vi "Apply Arm Motor Limits.vi"(8 "error in (no error)":errorcluster, 11 "KUKA youBot arm in":refnum<class "NI_Robotics_KUKA youBot Arm.lvclass">) -> (0 "error out":errorcluster, 3 "KUKA youBot arm out":refnum<class "NI_Robotics_KUKA youBot Arm.lvclass">)   [LabVIEW 2017, in "NI_Robotics_KUKA youBot Host.lvlib" / "NI_Robotics_KUKA youBot Arm.lvclass"]
uses:
  <vilib>/robotics/KUKA youBot/Basic Device/Arm/NI_Robotics_KUKA youBot Arm.lvclass
  <vilib>/robotics/KUKA youBot/Basic Device/Arm/NI_Robotics_KUKA youBot Arm.lvclass/NI_Robotics_KUKA youBot Arm.ctl
  <vilib>/robotics/KUKA youBot/Motor/Arm Motor/NI_Robotics_KUKA youBot Arm Motor.lvclass
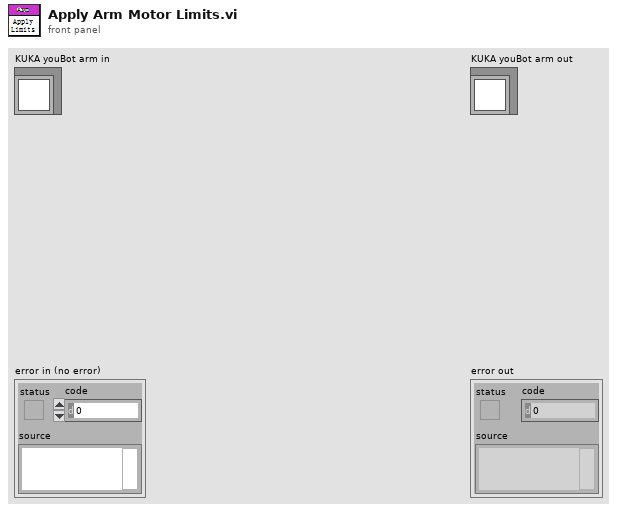
[diagram p1: front panel]
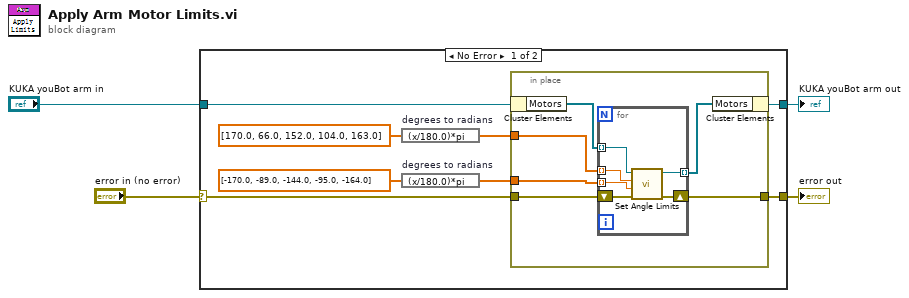
[diagram p0: block diagram]
diagram:
  n1 = case shown="No Error" "error in (no error)" {
    selector: "error in (no error)" -> [w11 w25]
    tunnel: [w10 w25] -> w3
    tunnel: [w9 w26] -> w1
    tunnel: "KUKA youBot arm in" -> [w12 w26]
    frame No Error {
      n2 = expression code="(x/180.0)*pi" "degrees to radians"(dbl[] [170.0, 66.0, 152.0, 104.0, 163.0]) -> (w6:dbl[])
      n3 = expression code="(x/180.0)*pi" "degrees to radians"(dbl[] [-170.0, -89.0, -144.0, -95.0, -164.0]) -> (w5:dbl[])
      n4 = in-place {
        in-place-border: w11 -> [w16]
        in-place-border: [w15] -> w10
        in-place-border: w6 -> [w14]
        in-place-border: w5 -> [w13]
        n5 = in-place-cluster #1(w12) -> ("Motors"=w18:refnum<class "NI_Robotics_KUKA youBot Arm Motor.lvclass">[])
        n6 = for {
          tunnel: w18 -> [w24] mode=indexing
          tunnel: [w23] -> w17 mode=indexing
          shift-right: [w21] -> w15
          shift-left: w16 -> [w22]
          tunnel: w14 -> [w20] mode=indexing
          tunnel: w13 -> [w19] mode=indexing
          n7 = call <vilib>:"Set Angle Limits.vi"("error in (no error)"=w22, "min angle (rad)"=w19, "max angle (rad)"=w20, "KUKA youBot arm motor in"=w24) -> ("error out"=w21:errorcluster, "KUKA youBot arm motor out"=w23:refnum<class "NI_Robotics_KUKA youBot Arm Motor.lvclass">)  [unwired: 6 in]
        }
        n8 = in-place-cluster #1("Motors"=w17) -> (w9:refnum<class "NI_Robotics_KUKA youBot Arm.lvclass">)
      }
    }
    frame Error {
    }
  }
  "error out" <- w3
  "KUKA youBot arm out" <- w1
